vi "postSubDataUE.vi"(6 "newValue (T)":bool=TRUE, 8 "error in (no error)":errorcluster, 9 "value":variant, 10 "subDataSV":T1, 11 "ViewThisComponent in":refnum<class "ViewThisComponent.lvclass">) -> (0 "error out":errorcluster, 3 "ViewThisComponent out":refnum<class "ViewThisComponent.lvclass">)   [LabVIEW 2016, in "ViewThisComponent.lvclass"]
uses:
  ViewThisComponent.lvclass
  Typedefs/SubDataSignal.ctl
  ViewThisComponent.lvclass/ViewThisComponent.ctl
  PubSubDataEvent/PubSubDataEvent.lvclass
  Typedefs/EXATypedefs.lvlib
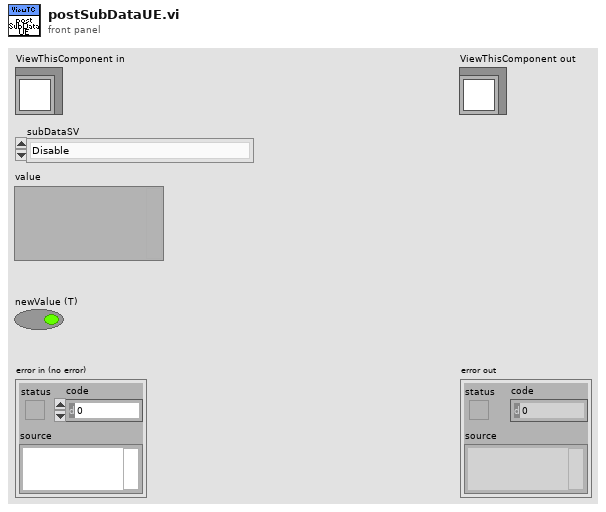
[diagram p1: front panel]
types:
  T1 = typedef "EXATypedefs.lvlib/SubDataSignal.ctl" = enum16{"Disable", "Enable", "Exit", "GoToStandby", "HeartbeatIn", "Start"}
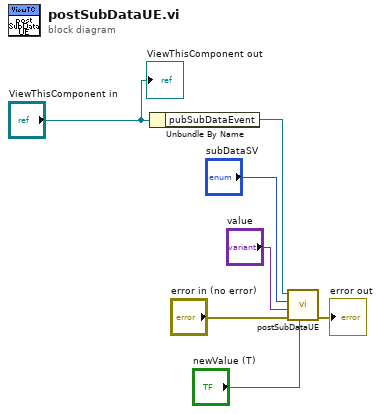
[diagram p0: block diagram]
diagram:
  n1 = Unbundle By Name("ViewThisComponent in") -> ("pubSubDataEvent"=w6:refnum<class "PubSubDataEvent.lvclass">)
  n2 = call "postSubDataUE.vi"("newValue (T)"="newValue (T)", "error in (no error)"="error in (no error)", "value"="value", "subDataSV"="subDataSV", "PubSubDataEvent in"=w6) -> ("error out"=→"error out":errorcluster)  [unwired: 5 in, 1 out]
  "ViewThisComponent out" <- "ViewThisComponent in"
